vi "Edit_Template_File.vi"(0 "Mode":T3(ring), 7 "Template Filename":path, 11 "Data Files":path[](array[path])) -> (4 "Cancelled":bool, 6 "Template Filename Out":path)   [LabVIEW 2022 SP3]
uses:
  Anemometry/Anemometry Sub Vis/Data_plotting_vis/File_Template_Clus.ctl
  Dispose_Channel.ctl
  Anemometry/Anemometry Sub Vis/Controls/Global_mode.ctl
panel:
  in  "Cancelled":bool
  out "index of element":i32
  in  "Add New Channel Named":bool
  in  "Edit Maths Equation":bool
  out "Current Case Name":string
  in  "Organise Channels":bool
  in  "Add New Channels Fr File":bool
  in  "OK":bool
  in  "Search String":string
  in  "Listbox":i32(listbox)
  out "Channel Name":string
  in  "Cluster":T1 {"Tolerance" min=0.0 format="%#.4f"}
  # "> 20  or  <20  or  =hello   or \n£hello  (not equal to hello)"
  # "<<Characters_to_Match>>  <<Replace_Whole_String_with_this>>"
  # "<<Channel_Name>> contains <<Characters to match>> or\n<<Channel_Name>> does not contain <<Characters to match>>"
  # "<<Channel_Name_A>> + <<Channel_Name_B>> or\nConcatenate <<Channel_Name_A>> and <<Channel_Name_B>>"
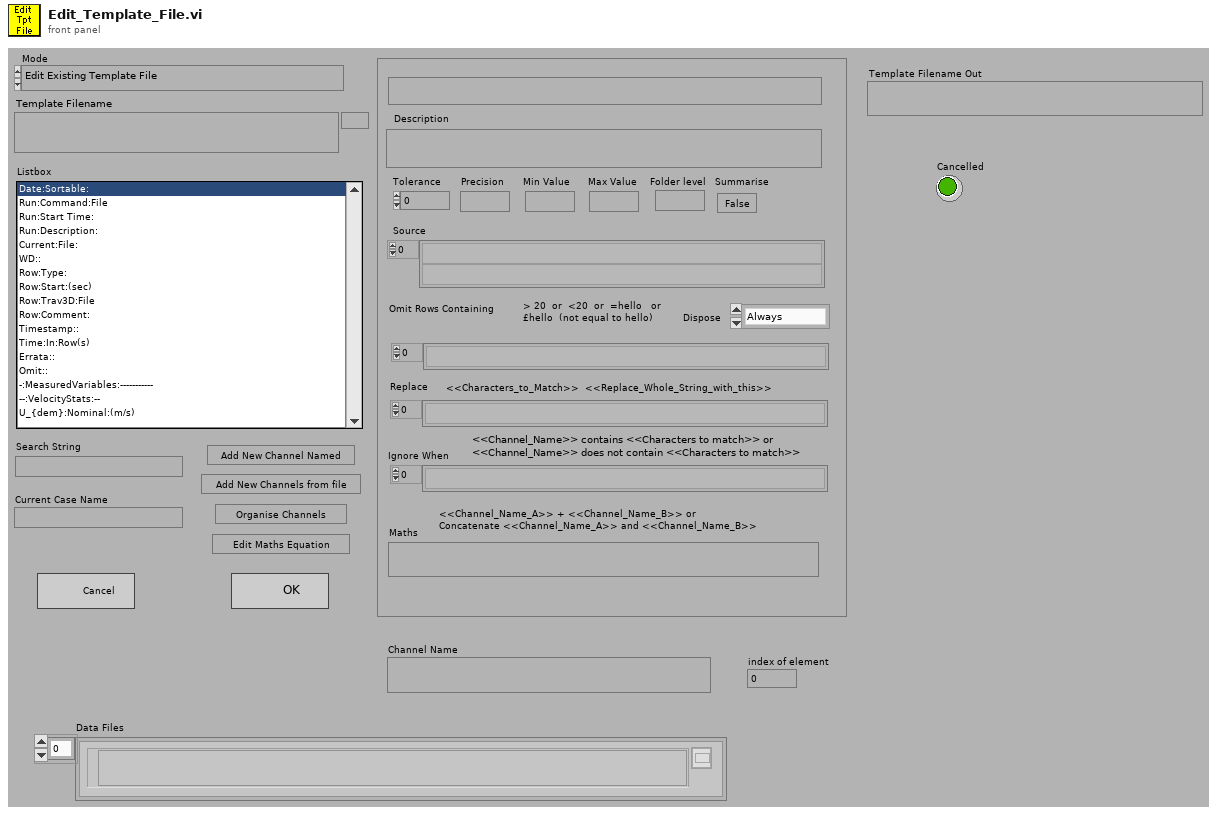
[diagram p1: front panel]
types:
  T1 = typedef "File_Template_Clus.ctl" = cluster{"Template Channel Name":string, "Description":string, "Tolerance":dbl, "Precision":string, "Folder level":string, "Source":string[], "Replace":string[], "Summarise":bool, "Min Value":string, "Maths":string, "Omit Rows Containing":string[], "Ignore When":string[], "Max Value":string, "Dispose":T2}
  T2 = typedef "Dispose_Channel.ctl" = enum16{"Always", "If Blank", "Never"}
  T3 = enum16{"Edit Existing Template File", "Create New Template File"}
  T4 = typedef "Global_mode.ctl" = enum16{"Read Global", "Load Global From File", "Write Global to File"}
  T5 = enum16{"Read Channels From File", "Read Channels from Server"}
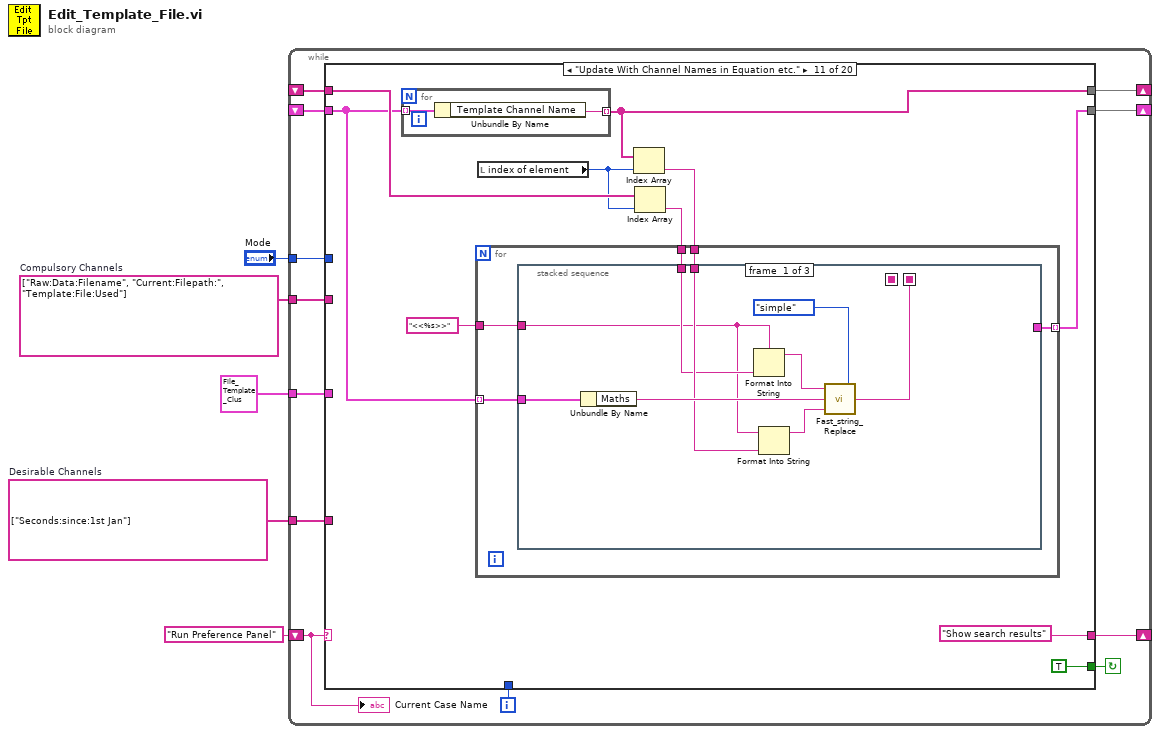
[diagram p0: block diagram]
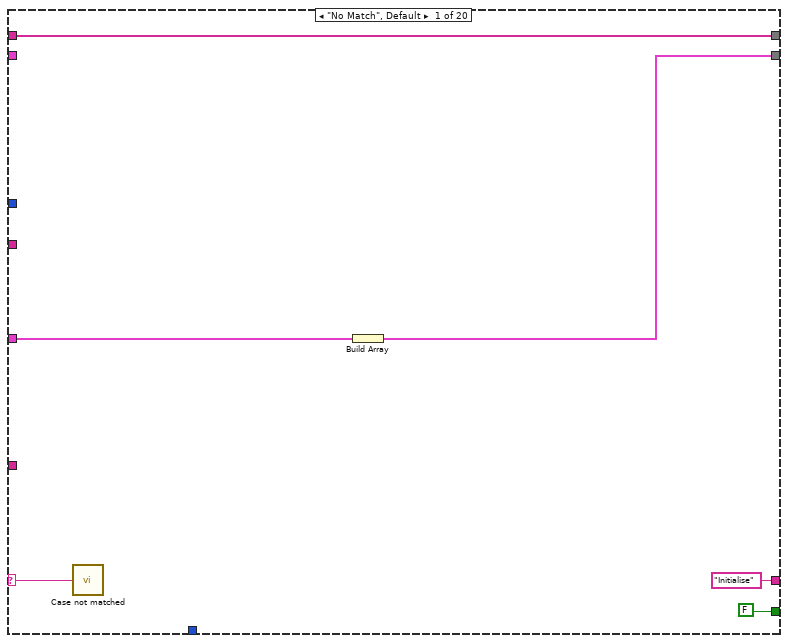
[diagram p2: hidden frame]
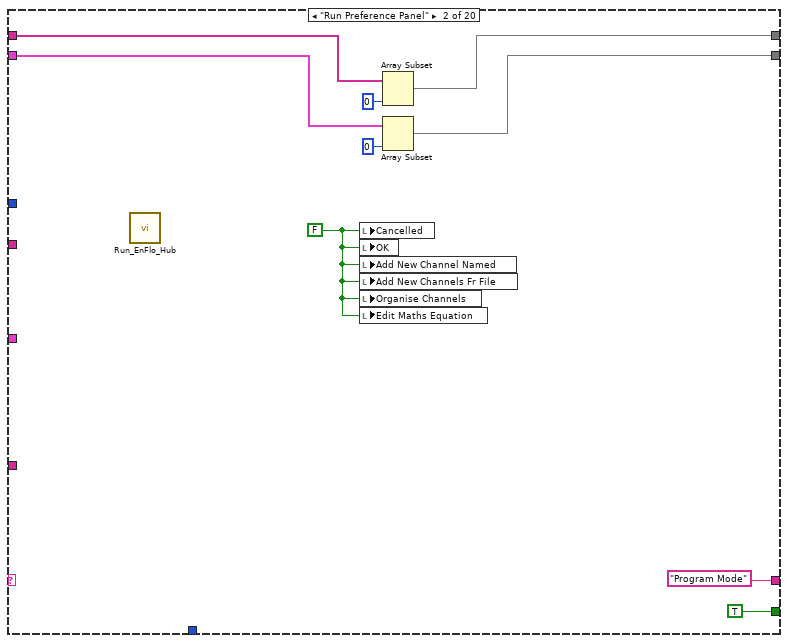
[diagram p3: hidden frame]
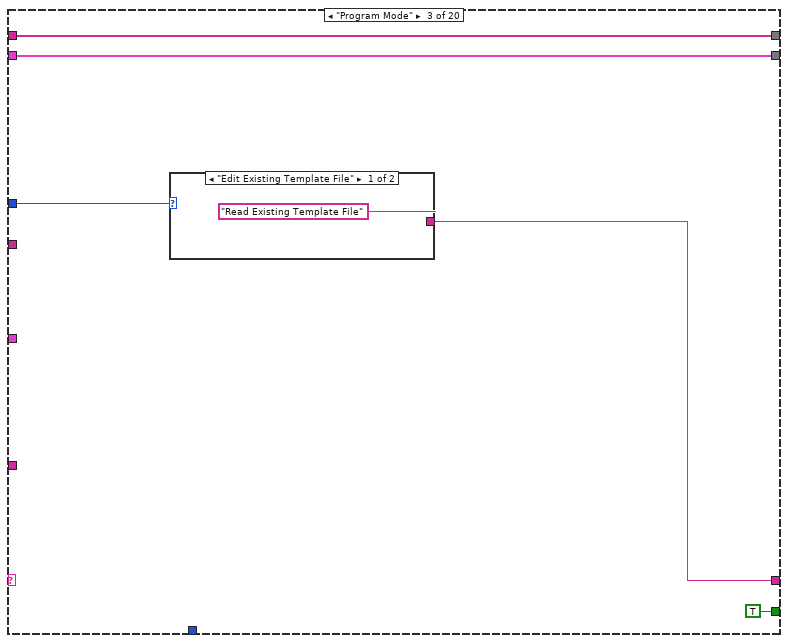
[diagram p4: hidden frame]
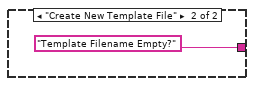
[diagram p5: hidden frame]
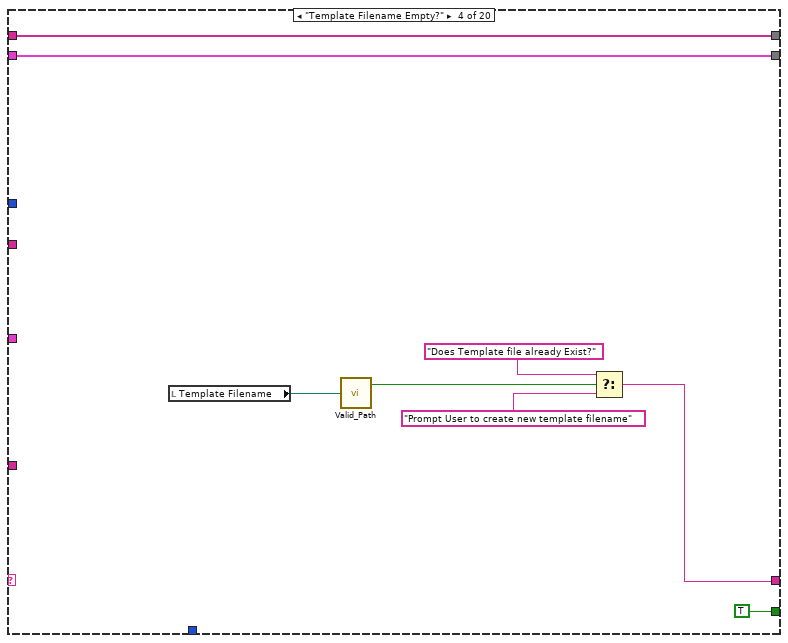
[diagram p6: hidden frame]
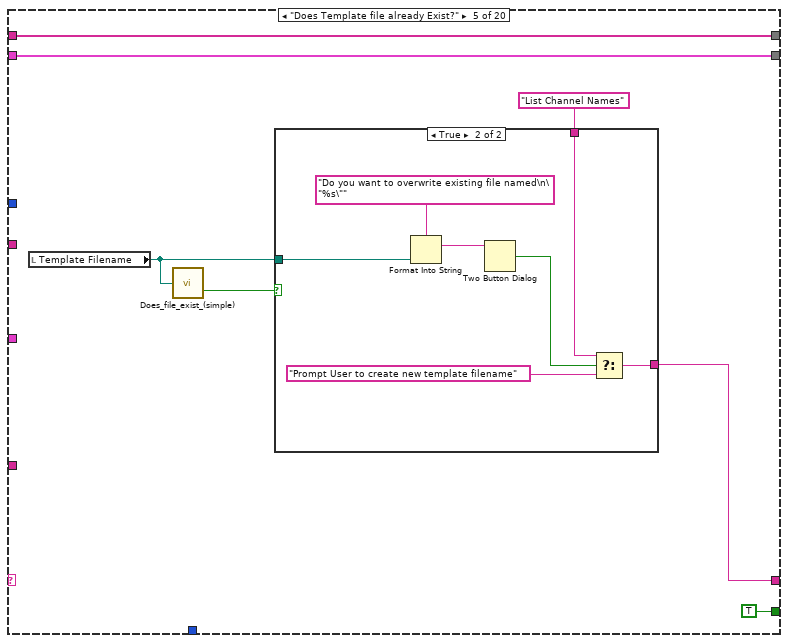
[diagram p7: hidden frame]
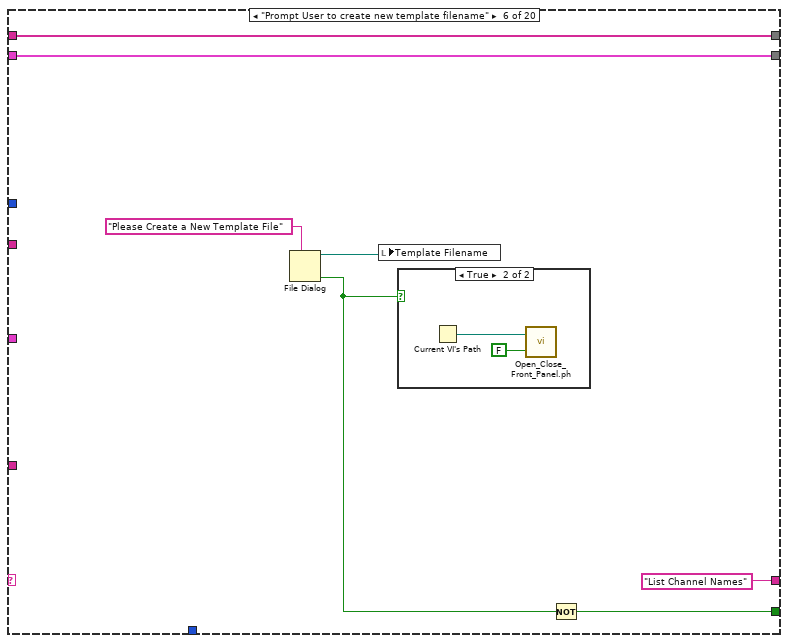
[diagram p9: hidden frame]
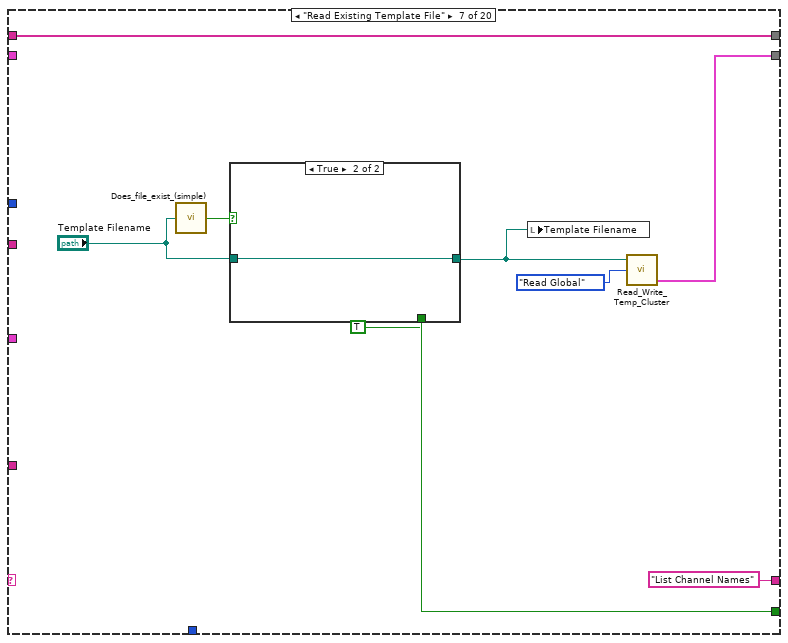
[diagram p11: hidden frame]
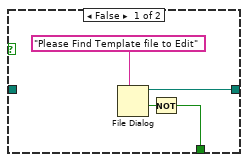
[diagram p12: hidden frame]
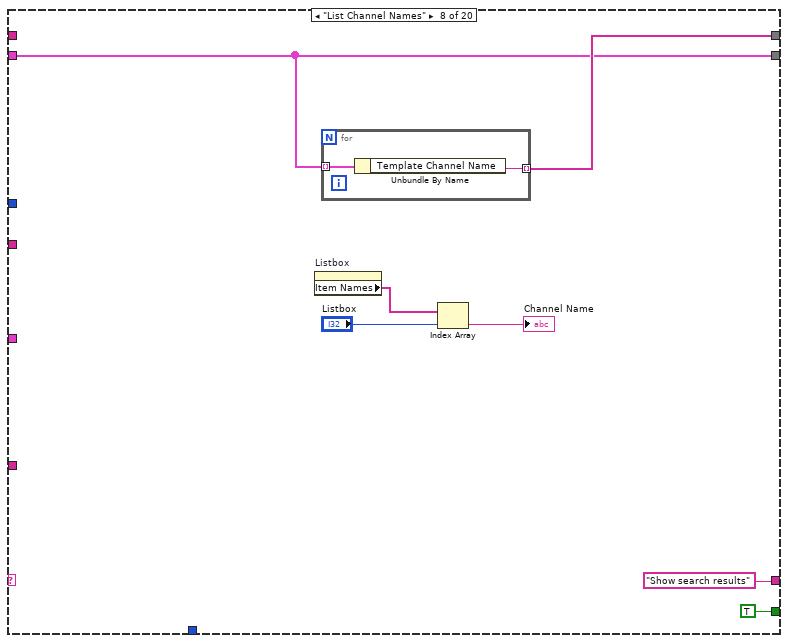
[diagram p13: hidden frame]
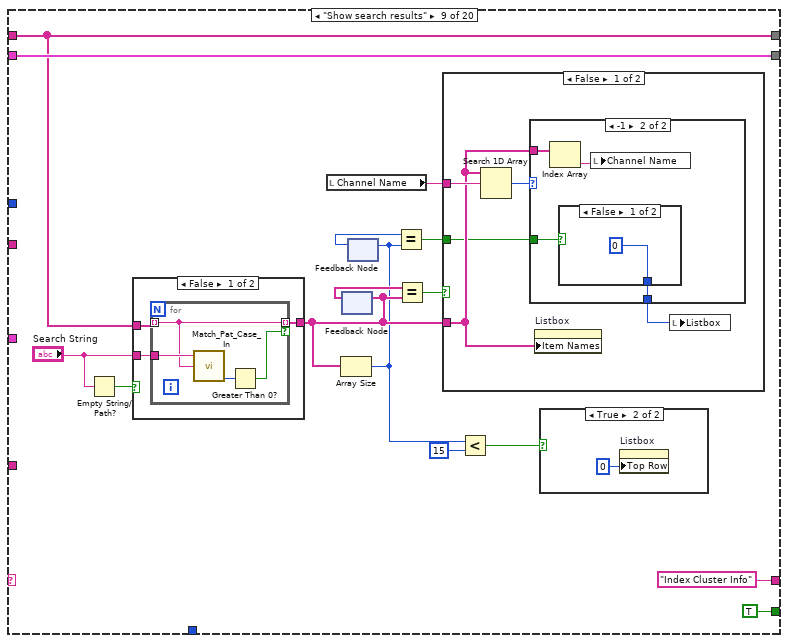
[diagram p14: hidden frame]
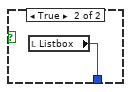
[diagram p17: hidden frame]
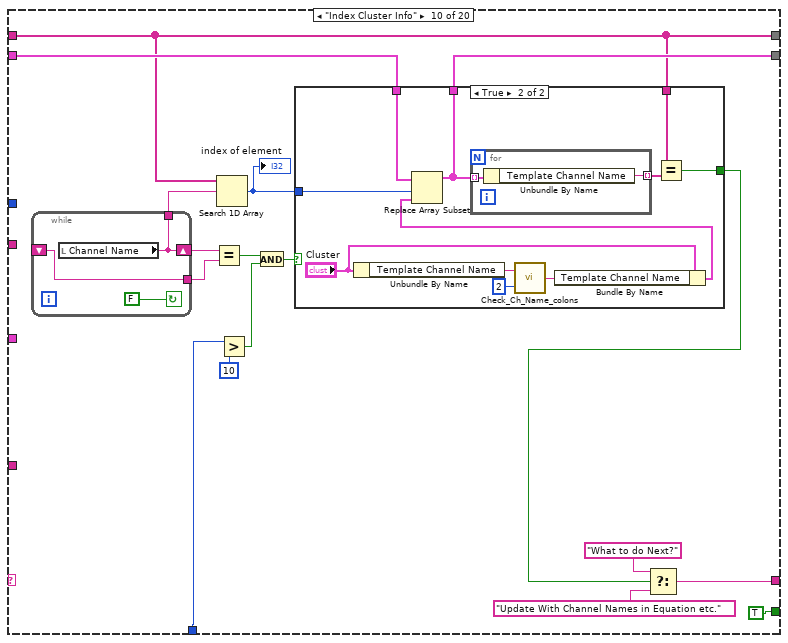
[diagram p20: hidden frame]
diagram:
  w1 = string[] ["Seconds:since:1st Jan"]  # Desirable Channels
  w2 = string[] ["Raw:Data:Filename", "Current:Filepath:", "Template:File:Used"]  # Compulsory Channels
  n1 = while {
    tunnel: T1 {"Template Channel Name"="", "Description"="", "Tolerance"=0.0, "Precision"="", "Folder level"="", "Source"=[], "Replace"=[], "Summarise"=FALSE, "Min Value"="", "Maths"="", "Omit Rows Containing"=[], "Ignore When"=[], "Max Value"="", "Dispose"=enum."Never"} ("Cluster") -> [w11]
    shift-left: _ -> [w12]
    shift-right: [w13] -> _
    tunnel: "Mode" -> [w15]
    shift-left: _ -> [w8]
    shift-right: [w14] -> _
    shift-left: "Run Preference Panel" -> [w10]
    shift-right: [w16] -> _
    tunnel: w2 -> [w7]
    tunnel: w1 -> [w6]
    i -> [w9]
    stop <- w17 continue-if-true
    n2 = case shown="\"Update With Channel Names in Equation etc.\"" w10 {
      selector: w10 -> [w18 _ _ _ _ _ _ _ _ _ _ _ _ _ _ _ _ _ _ _]
      tunnel: [FALSE TRUE TRUE TRUE TRUE w64 w72 TRUE TRUE TRUE TRUE TRUE TRUE TRUE TRUE TRUE TRUE TRUE TRUE FALSE] -> w17
      tunnel: ["Initialise" "Program Mode" w33 w44 w49 "List Channel Names" ("t") "List Channel Names" "Show search results" "Index Cluster Info" w138 "Show search results" "Update cluster info after edit" "Update cluster info after edit" "Update cluster info after edit" "Save Template File" ("t") w301 "Check Tolerance and Precision" "Save Template File" w432 "End" ("t")] -> w16
      tunnel: w15 -> [_ _ w36 _ _ _ _ _ _ _ _ _ _ _ _ _ _ _ _ _]
      tunnel: [w19 w25 w34 w45 w52 w68 w75 w89 w105 w141 w174 w214 w255 w272 w296 w319 w324 w384 w427 w450] -> w14
      tunnel: w8 -> [_ w26 w34 w45 w52 w68 _ w89 w105 w145 w173 w216 w256 w277 w296 w319 w335 w388 w427 w450]
      tunnel: [w21 w28 w35 w46 w53 w69 w74 w91 w104 w137 w175 w215 w257 w279 w298 w320 w331 w385 w436 w451] -> w13
      tunnel: w12 -> [w21 w29 w35 w46 w53 w69 w74 _ w104 w137 w176 w217 w258 w279 w298 w320 w332 w385 w436 w451]
      tunnel: w11 -> [w20 _ _ _ _ _ _ _ _ _ _ w213 _ _ _ _ w322 _ _ _]
      tunnel: w9 -> [_ _ _ _ _ _ _ _ _ w135 _ _ _ _ _ _ _ _ _ _]
      tunnel: w7 -> [_ _ _ _ _ _ _ _ _ _ _ _ _ _ _ _ w328 _ _ _]
      tunnel: w6 -> [_ _ _ _ _ _ _ _ _ _ _ _ _ _ _ _ w325 _ _ _]
      frame "No Match", Default {
        n3 = call "Case not matched.vi"("Case Name not Matched"=w18) -> ()
        n4 = Build Array(w20) -> (w19:T1[])
      }
      frame "Run Preference Panel" {
        w24 = FALSE ("Add channel Fr Results File")
        n5 = call "Run_EnFlo_Hub.vi"() -> ()  [unwired: 1 in, 7 out]
        n6 = local write "Cancelled"(w24) -> ()
        n7 = local write "OK"(w24) -> ()
        n8 = local write "Add New Channel Named"(w24) -> ()
        n9 = local write "Add New Channels Fr File"(w24) -> ()
        n10 = local write "Organise Channels"(w24) -> ()
        n11 = local write "Edit Maths Equation"(w24) -> ()
        n12 = Array Subset(array=w29, length=0 ("Array Length")) -> (w28:string[])  [unwired: 1 in]
        n13 = Array Subset(array=w26, length=0 ("Array Length")) -> (w25:T1[])  [unwired: 1 in]
      }
      frame "Program Mode" {
        n14 = case shown="\"Edit Existing Template File\"" w36 {
          tunnel: ["Read Existing Template File" "Template Filename Empty?"] -> w33
          frame "Edit Existing Template File" {
          }
          frame "Create New Template File" {
          }
        }
      }
      frame "Template Filename Empty?" {
        n15 = local read "Template Filename"() -> (w43:path)
        n16 = call "Valid_Path.vi"("Filename"=w43) -> ("Valid Path?"=w42:bool)
        n17 = Select(t="Does Template file already Exist?", s=w42, f="Prompt User to create new template filename" ("t")) -> (s? t:f=w44:string)
      }
      frame "Does Template file already Exist?" {
        n18 = local read "Template Filename"() -> (w50:path)
        n19 = call "Does_file_exist_(simple).vi"("Pathname"=w50) -> ("exists?"=w51:bool)
        n20 = case shown="True" w51 {
          tunnel: w50 -> [_ w62]
          tunnel: [w55 w57] -> w49
          tunnel: "List Channel Names" ("t") -> [w55 w56]
          frame False {
          }
          frame True {
            n21 = Format Into String(format string="Do you want to overwrite existing file named\n\"%s\"" ("Format String"), w62) -> (resulting string=w60:string)  [unwired: 2 in, 1 out]
            n22 = Two Button Dialog(message=w60) -> (T button?=w58:bool)  [unwired: 2 out]
            n23 = Select(t=w56, s=w58, f="Prompt User to create new template filename") -> (s? t:f=w57:string)
          }
        }
      }
      frame "Prompt User to create new template filename" {
        n24 = File Dialog(7:"Please Create a New Template File" ("prompt")) -> (1:w63:bool, 3:w67:path)  [unwired: 1 in, 7 out]
        n25 = local write "Template Filename"(w67) -> ()
        n26 = case shown="True" w63 {
          frame False {
          }
          frame True {
            n27 = Current VI's Path() -> (path=w71:path)
            n28 = call "Open_Close_Front_Panel.ph.vi"("openWindow (T)"=FALSE ("Front Panel Window:Open"), "VI path"=w71) -> ()  [unwired: 1 in, 1 out]
          }
        }
        n29 = Not(x=w63) -> (.not. x?=w64:bool)
      }
      frame "Read Existing Template File" {
        n30 = call "Does_file_exist_(simple).vi"("Pathname"="Template Filename") -> ("exists?"=w78:bool)
        n31 = case shown="True" w78 {
          tunnel: [w83 w85] -> w73
          tunnel: "Template Filename" -> [_ w85]
          tunnel: [w80 TRUE] -> w72
          frame False {
            n32 = File Dialog(7:"Please Find Template file to Edit" ("prompt")) -> (1:w81:bool, 3:w83:path)  [unwired: 1 in, 7 out]
            n33 = Not(x=w81) -> (.not. x?=w80:bool)
          }
          frame True {
          }
        }
        n34 = local write "Template Filename"(w73) -> ()
        n35 = call "Read_Write_Temp_Cluster.vi"("Mode"=Global_mode."Read Global", "Template File"=w73) -> ("Template Info Array Out"=w75:T1[])  [unwired: 1 in, 2 out]
      }
      frame "List Channel Names" {
        n36 = property on="Listbox" class="LstBox (strict)"() -> ("Item Names"=w88:string[])  [unwired: 2 in, 2 out]
        n37 = for {
          tunnel: w89 -> [w94] mode=indexing
          tunnel: [w93] -> w91 mode=indexing
          n38 = Unbundle By Name(w94) -> ("Template Channel Name"=w93:string)
        }
        n39 = Index Array(array=w88, index="Listbox") -> (element=→"Channel Name":string)
      }
      frame "Show search results" {
        n40 = Empty String/Path?(string/path="Search String") -> (empty?=w107:bool)
        n41 = case shown="False" w107 {
          tunnel: "Search String" -> [w125 _]
          tunnel: w104 -> [w124 w130]
          tunnel: [w123 w130] -> w100
          frame False {
            n42 = for {
              tunnel: w125 -> [w129]
              tunnel: w124 -> [w127] mode=indexing
              tunnel: [w127] -> w123 mode=indexing if=w126
              n43 = call "Match_Pat_Case_In.vi"("String to match"=w129, "String"=w127) -> ("offset past match"=w128:i32)  [unwired: 1 in, 3 out]
              n44 = Greater Than 0?(x=w128) -> (x > 0?=w126:bool)
            }
          }
          frame True {
          }
        }
        n45 = local read "Channel Name"() -> (w101:string)
        n46 = Array Size(array=w100) -> (size(s)=w97:i32)
        n47 = feedback-in #1(w100) -> ()
        n48 = feedback #1() -> (w103:string[])  [unwired: 1 in]
        n49 = feedback #2() -> (w99:i32)  [unwired: 1 in]
        n50 = feedback-in #2(w97) -> ()
        n51 = Equal?(x=w99, y=w97) -> (x = y?=w98:bool)
        n52 = Equal?(x=w103, y=w100) -> (x = y?=w102:bool)
        n53 = case shown="False" w102 {
          tunnel: w100 -> [w113 _]
          tunnel: w101 -> [w115 _]
          tunnel: w98 -> [w112 _]
          frame False {
            n54 = Search 1D Array(1D array=w113, element=w115) -> (index of element=w114:i32)  [unwired: 1 in]
            n55 = case shown="-1" w114 {
              selector: w114 -> [w116 _]
              tunnel: w113 -> [_ w120]
              tunnel: w112 -> [_ w118]
              tunnel: [w116 w117] -> w111
              frame Default {
              }
              frame -1 {
                n56 = Index Array(array=w120) -> (element=w119:string)  [unwired: 1 in]
                n57 = case shown="False" w118 {
                  tunnel: [0 ("Listbox") w122] -> w117
                  frame False {
                  }
                  frame True {
                    n58 = local read "Listbox"() -> (w122:i32)
                  }
                }
                n59 = local write "Channel Name"(w119) -> ()
              }
            }
            n60 = property on="Listbox" class="LstBox (strict)"("Item Names"=w113) -> ()  [unwired: 2 in, 2 out]
            n61 = local write "Listbox"(w111) -> ()
          }
          frame True {
          }
        }
        n62 = Less?(x=w97, y=15) -> (x < y?=w95:bool)
        n63 = case shown="True" w95 {
          frame False {
          }
          frame True {
            n64 = property on="Listbox" class="LstBox (strict)"("Top Row"=0) -> ()  [unwired: 2 in, 2 out]
          }
        }
      }
      frame "Index Cluster Info" {
        n65 = while {
          tunnel: [w149] -> w142
          tunnel: [w150] -> w143
          shift-left: _ -> [w150]
          shift-right: [w149] -> w144
          stop <- FALSE continue-if-true
          n66 = local read "Channel Name"() -> (w149:string)
        }
        n67 = Equal?(x=w144, y=w143) -> (x = y?=w133:bool)
        n68 = Search 1D Array(1D array=w137, element=w142) -> (index of element=w146:i32)  [unwired: 1 out]
        "index of element" <- w146
        n69 = Greater?(x=w135, y=10) -> (0:w132:bool)
        n70 = And(x=w133, y=w132) -> (x .and. y?=w131:bool)
        n71 = case shown="True" w131 {
          tunnel: w146 -> [w154 w164]
          tunnel: w145 -> [w152 w165]
          tunnel: [w152 w161] -> w141
          tunnel: w137 -> [_ w162]
          tunnel: [TRUE w160] -> w136
          frame False {
            n72 = Index Array(array=w152, index=w154) -> (element=w153:T1)
            n73 = local write "Cluster"(w153) -> ()
          }
          frame True {
            n74 = Unbundle By Name("Cluster") -> ("Template Channel Name"=w158:string)
            n75 = call "Check_Ch_Name_colons.vi"("No of Colons"=2, "Ch Name in"=w158) -> ("Ch Name out"=w157:string)
            n76 = Bundle By Name(cluster="Cluster", "Template Channel Name"=w157) -> (w155:T1)
            n77 = Replace Array Subset(array=w165, new element=w155, index=w164) -> (w161:T1[])
            n78 = for {
              tunnel: w161 -> [w167] mode=indexing
              tunnel: [w166] -> w163 mode=indexing
              n79 = Unbundle By Name(w167) -> ("Template Channel Name"=w166:string)
            }
            n80 = Equal?(x=w162, y=w163) -> (x = y?=w160:bool)
          }
        }
        n81 = Select(t="What to do Next?", s=w136, f="Update With Channel Names in Equation etc.") -> (s? t:f=w138:string)
      }
      frame "Update With Channel Names in Equation etc." {
        n82 = for {
          tunnel: w173 -> [w210] mode=indexing
          tunnel: [w209] -> w175 mode=indexing
          n83 = Unbundle By Name(w210) -> ("Template Channel Name"=w209:string)
        }
        n84 = local read "index of element"() -> (w171:i32)
        n85 = Index Array(array=w175, index=w171) -> (element=w169:string)
        n86 = Index Array(array=w176, index=w171) -> (element=w170:string)
        n87 = for {
          tunnel: w173 -> [w180] mode=indexing
          tunnel: w169 -> [w182]
          tunnel: [w179] -> w174 mode=indexing
          tunnel: w170 -> [w181]
          tunnel: "<<%s>>" ("Format String") -> [w178]
          n88 = stacked-sequence {
            seq-local: [w185 _ _] -> [_ _ w208]
            seq-local: [_ w193 _] -> [_ _ w206]
            tunnel: w180 -> [w191 w197 w205]
            tunnel: w182 -> [w189 w195 _]
            tunnel: w181 -> [w186 w194 _]
            tunnel: [_ _ w207] -> w179
            tunnel: w178 -> [w184 w192 _]
            frame #0 {
              n89 = Unbundle By Name(w191) -> ("Maths"=w190:string)
              n90 = Format Into String(format string=w184, w186) -> (resulting string=w187:string)  [unwired: 2 in, 1 out]
              n91 = Format Into String(format string=w184, w189) -> (resulting string=w188:string)  [unwired: 2 in, 1 out]
              n92 = call "Fast_string_Replace.vi"("mode"=enum16{"simple", "regex"}."simple", "Replace match with:"=w188, "Input String"=w190, "matchThis"=w187) -> ("Output String"=w185:string)  [unwired: 1 out]
            }
            frame #1 {
              n93 = Unbundle By Name(w197) -> ("Ignore When"=w196:string[])
              n94 = for {
                tunnel: w196 -> [w204] mode=indexing
                tunnel: w195 -> [w203]
                tunnel: w194 -> [w200]
                tunnel: [w199] -> w193 mode=indexing
                tunnel: w192 -> [w198]
                n95 = Format Into String(format string=w198, w200) -> (resulting string=w201:string)  [unwired: 2 in, 1 out]
                n96 = Format Into String(format string=w198, w203) -> (resulting string=w202:string)  [unwired: 2 in, 1 out]
                n97 = call "Fast_string_Replace.vi"("Replace match with:"=w202, "Input String"=w204, "matchThis"=w201) -> ("Output String"=w199:string)  [unwired: 1 in, 1 out]
              }
            }
            frame #2 {
              n98 = Bundle By Name(cluster=w205, "Maths"=w208, "Ignore When"=w206) -> (w207:T1)
            }
          }
        }
      }
      frame "Select New Channel" {
        n99 = local read "Add New Channel Named"() -> (w212:bool)
        n100 = case shown="False" w212 {
          tunnel: [w223 w227] -> w218
          tunnel: [FALSE ("Add channel Fr Results File") FALSE ("Add channel Fr Results File")] -> w211
          frame False {
            n101 = call "Select_a_Channel.vi"("Mode"=T5."Read Channels From File", "Data Files"="Data Files") -> ("Selected Channel Names"=w223:string[])  [unwired: 1 in, 5 out]
          }
          frame True {
            n102 = call "Input_String_Dialog.vi"("Message to user"="Enter New Channel Name") -> ("Ok Out"=w229:bool, "Output string"=w230:string)  [unwired: 1 in]
            n103 = Build Array(w230) -> (w228:string[])
            n104 = Select(t=w228, s=w229, f=string[] []) -> (s? t:f=w227:string[])
          }
        }
        n105 = for {
          tunnel: w218 -> [w236] mode=indexing
          shift-right: [w234] -> w215
          shift-left: w217 -> [w235]
          shift-right: [w237] -> w214
          shift-left: w216 -> [w238]
          tunnel: w213 -> [w240]
          n106 = Build Array(w236) -> (w243:string[])
          n107 = while {
            tunnel: [w244] -> w233
            tunnel: w236 -> [w246]
            tunnel: w235 -> [w247]
            i -> [w245]
            stop <- w248 continue-if-true
            n108 = case shown="1, Default" w245 {
              selector: w245 -> [_ w251]
              tunnel: [w250 w253] -> w244
              tunnel: w246 -> [w250 w252]
              frame 0 {
              }
              frame 1, Default {
                n109 = Format Into String(format string="%s_DUPLICATE%d" ("Format String"), w252, w251) -> (resulting string=w253:string)  [unwired: 2 in, 1 out]
              }
            }
            n110 = Search 1D Array(1D array=w247, element=w244) -> (index of element=w249:i32)  [unwired: 1 out]
            n111 = Greater Or Equal To 0?(x=w249) -> (x >= 0?=w248:bool)
          }
          n112 = Bundle By Name(cluster=w240, "Template Channel Name"=w233, "Source"=w243, "Summarise"=FALSE ("Bundle Element"), "Dispose"=Dispose_Channel."If Blank", "Tolerance"=1.0 ("Bundle Element")) -> (w239:T1)
          n113 = Build Array (concatenate)(w238, w239) -> (w237:T1[])
          n114 = Build Array (concatenate)(w235, w233) -> (w234:string[])
        }
        n115 = local write "Add New Channel Named"(w211) -> ()
        n116 = local write "Add New Channels Fr File"(w211) -> ()
      }
      frame "Organise Channels" {
        n117 = call "Organise_String_Array.vi"("Input Array"=w258) -> ("Output Array"=w257:string[])
        n118 = for {
          tunnel: w258 -> [w266]
          tunnel: w257 -> [w265] mode=indexing
          tunnel: w256 -> [w263]
          tunnel: [w262] -> w255 mode=indexing
          n119 = Search 1D Array(1D array=w266, element=w265) -> (index of element=w264:i32)  [unwired: 1 out]
          n120 = Index Array(array=w263, index=w264) -> (element=w262:T1)
        }
        n121 = local write "Organise Channels"(FALSE ("Add channel Fr Results File")) -> ()
      }
      frame "Edit Maths Equation" {
        n122 = property on="Listbox" class="LstBox (strict)"() -> ("Item Names"=w269:string[])  [unwired: 2 in, 2 out]
        n123 = local read "Listbox"() -> (w280:i32)
        n124 = Index Array(array=w269, index=w280) -> (element=w278:string)
        n125 = Search 1D Array(1D array=w279, element=w278) -> (index of element=w274:i32)  [unwired: 1 out]
        n126 = Index Array(array=w277, index=w274) -> (element=w273:T1)
        n127 = Unbundle By Name(w273) -> ("Template Channel Name"=w276:string, "Maths"=w275:string)
        n128 = local write "Edit Maths Equation"(FALSE ("Add channel Fr Results File")) -> ()
        n129 = call "Edit_Maths_Equation.vi"("Template Info Array"=w277, "Maths Equation In"=w275, "Channel Name"=w276) -> ("Template Info Array Out"=w271:T1[], "Maths Equation Out"=w268:string)  [unwired: 1 out]
        n130 = Empty String/Path?(string/path=w268) -> (empty?=w267:bool)
        n131 = case shown="False" w267 {
          tunnel: w269 -> [w285 _]
          tunnel: w268 -> [w284 _]
          frame False {
            w286 = TRUE  # Dialog Box (T)
            n132 = call "Do_channel_mathsPLL.vi"("Channel Names"=w285, "Maths Equation"=w284) -> ("Error String"=w290:string)  [unwired: 3 in, 2 out]
            n133 = Empty String/Path?(string/path=w290) -> (empty?=w292:bool)
            n134 = Not(x=w292) -> (.not. x?=w289:bool)
            n135 = Bundle By Name(cluster=errorcluster {"status"=FALSE, "code"=0, "source"=""} ("error in (no error)"), "source"=w290, "status"=w289) -> (w288:errorcluster)
            n136 = call "EnFlo_Error_Handler.vi"("error in (no error)"=w288, "Error Type"="Maths Equation", "Dialog Box (F)"=w286) -> ()  [unwired: 3 out]
          }
          frame True {
          }
        }
        n137 = Bundle By Name(cluster=w273, "Maths"=w268) -> (w270:T1)
        n138 = Replace Array Subset(array=w271, new element=w270, index=w274) -> (w272:T1[])
      }
      frame "Update cluster info after edit" {
        n139 = local read "Channel Name"() -> (w294:string)
        n140 = Search 1D Array(1D array=w298, element=w294) -> (index of element=w297:i32)  [unwired: 1 out]
        n141 = Index Array(array=w296, index=w297) -> (element=w295:T1)
        n142 = local write "Cluster"(w295) -> ()
      }
      frame "What to do Next?" {
        n143 = Select(t="Select New Channel", s="Add New Channels Fr File", f="List Channel Names") -> (s? t:f=w312:string)
        n144 = Select(t="Organise Channels", s="Organise Channels", f=w312) -> (s? t:f=w305:string)
        n145 = Select(t="Edit Maths Equation", s="Edit Maths Equation", f=w305) -> (s? t:f=w307:string)
        n146 = Select(t="Select New Channel", s="Add New Channel Named", f=w307) -> (s? t:f=w306:string)
        n147 = Select(t="Check Template File", s="OK", f=w306) -> (s? t:f=w302:string)
        n148 = Select(t="Close Panel", s="Cancelled", f=w302) -> (s? t:f=w301:string)
        "Cancelled" <- "Cancelled"
      }
      frame "Check Template File" {
        n149 = for {
          tunnel: w335 -> [w381] mode=indexing
          tunnel: [w380] -> w329 mode=indexing
          tunnel: [w379] -> w326 mode=indexing
          n150 = Unbundle By Name(w381) -> ("Template Channel Name"=w382:string)
          n151 = call "Check_Ch_Name_colons.vi"("No of Colons"=2, "Ch Name in"=w382) -> ("Ch Name out"=w379:string)
          n152 = Bundle By Name(cluster=w381, "Template Channel Name"=w379) -> (w380:T1)
        }
        n153 = for {
          tunnel: w328 -> [w360] mode=indexing
          tunnel: w326 -> [w362]
          tunnel: w322 -> [w359]
          tunnel: [w358] -> w330 mode=indexing if=w355
          shift-right: [w356] -> w327
          shift-left: w329 -> [w357]
          n154 = Search 1D Array(1D array=w362, element=w360) -> (index of element=w361:i32)  [unwired: 1 in]
          n155 = case shown="-1" w361 {
            selector: w361 -> [w364 _]
            tunnel: w360 -> [_ w375]
            tunnel: w359 -> [_ w376]
            tunnel: ["" ("Ch Name out") w375] -> w358
            tunnel: w357 -> [w365 w373]
            tunnel: [w363 w372] -> w356
            tunnel: [FALSE TRUE] -> w355
            frame Default {
              n156 = in-place {
                n157 = in-place-array #3(w365, w364) -> (w370:T1)
                n158 = Bundle By Name(cluster=w370, "Dispose"=Dispose_Channel."Never") -> (w369:T1)
                n159 = in-place-array #3(w369) -> (w363:T1[])  [unwired: 1 out]
              }
            }
            frame -1 {
              n160 = Bundle By Name(cluster=w376, "Template Channel Name"=w375, "Dispose"=Dispose_Channel."Never", "Summarise"=FALSE) -> (w374:T1)
              n161 = Build Array (concatenate)(w373, w374) -> (w372:T1[])
            }
          }
        }
        n162 = for {
          tunnel: w325 -> [w341] mode=indexing
          tunnel: w326 -> [w343]
          tunnel: [w340] -> w323 mode=indexing if=w337
          shift-right: [w338] -> w324
          shift-left: w327 -> [w339]
          tunnel: w322 -> [w336]
          n163 = Search 1D Array(1D array=w343, element=w341) -> (index of element=w342:i32)  [unwired: 1 in]
          n164 = case shown="-1" w342 {
            tunnel: w341 -> [_ w352]
            tunnel: ["" ("Ch Name out") w352] -> w340
            tunnel: w339 -> [w344 w350]
            tunnel: [w344 w349] -> w338
            tunnel: [FALSE TRUE] -> w337
            tunnel: w336 -> [_ w347]
            frame Default {
            }
            frame -1 {
              n165 = Bundle By Name(cluster=w347, "Template Channel Name"=w352, "Dispose"=Dispose_Channel."Never", "Summarise"=FALSE) -> (w351:T1)
              n166 = Build Array (concatenate)(w350, w351) -> (w349:T1[])
            }
          }
        }
        n167 = Build Array (concatenate)(w332, w330, w323) -> (w331:string[])
      }
      frame "Check Tolerance and Precision" {
        n168 = for {
          tunnel: w388 -> [w391] mode=indexing
          tunnel: [w392] -> w384 mode=indexing
          n169 = Unbundle By Name(w391) -> ("Tolerance"=w389:dbl, "Precision"=w390:string)
          n170 = Empty String/Path?(string/path=w390) -> (empty?=w393:bool)
          n171 = case shown="False" w393 {
            tunnel: [w397 w425] -> w392
            tunnel: w391 -> [w396 w425]
            tunnel: w390 -> [w400 _]
            tunnel: w389 -> [w395 _]
            frame False {
              n172 = Fract/Exp String To Number(string=w400) -> (number=w394:dbl)  [unwired: 3 in, 1 out]
              n173 = Greater?(x=w395, y=0.7) -> (0:w398:bool)
              n174 = case shown="False" w398 {
                tunnel: [w402 w424] -> w397
                tunnel: w396 -> [w401 w424]
                tunnel: w395 -> [w406 _]
                tunnel: w394 -> [w403 _]
                frame False {
                  n175 = Greater?(x=w406, y=0.07) -> (0:w404:bool)
                  n176 = case shown="True" w404 {
                    tunnel: w403 -> [w410 w417]
                    tunnel: [w408 w419] -> w402
                    tunnel: w401 -> [w407 w418]
                    frame True {
                      n177 = Greater Than 0?(x=w410) -> (x > 0?=w409:bool)
                      n178 = case shown="False" w409 {
                        tunnel: [w412 w414] -> w408
                        tunnel: w407 -> [w413 w414]
                        frame False {
                          n179 = Bundle By Name(cluster=w413, "Precision"="1") -> (w412:T1)
                        }
                        frame True {
                        }
                      }
                    }
                    frame False {
                      n180 = Greater?(x=w417, y=1.0) -> (0:w415:bool)
                      n181 = case shown="False" w415 {
                        tunnel: [w421 w423] -> w419
                        tunnel: w418 -> [w422 w423]
                        frame False {
                          n182 = Bundle By Name(cluster=w422, "Precision"="2") -> (w421:T1)
                        }
                        frame True {
                        }
                      }
                    }
                  }
                }
                frame True {
                }
              }
            }
            frame True {
            }
          }
        }
      }
      frame "Save Template File" {
        n183 = local read "Template Filename"() -> (w428:path)
        "Template Filename Out" <- w428
        n184 = call "Does_file_exist_(simple).vi"("Pathname"=w428) -> ("exists?"=w429:bool)
        n185 = case shown="True" w429 {
          tunnel: w427 -> [_ w440]
          tunnel: [TRUE w438] -> w426
          tunnel: w428 -> [_ w439]
          frame False {
          }
          frame True {
            n186 = call "Read_Write_Temp_Cluster.vi"("Mode"=Global_mode."Read Global", "Template File"=w439) -> ("Template Info Array Out"=w441:T1[])  [unwired: 1 in, 2 out]
            n187 = Not Equal?(x=w441, y=w440) -> (x != y?=w438:bool)
          }
        }
        n188 = local write "Mode"(T3."Edit Existing Template File" ("Mode")) -> ()
        n189 = case shown="True" w426 {
          tunnel: w428 -> [_ w444]
          tunnel: w427 -> [_ w443]
          frame False {
          }
          frame True {
            n190 = call "Read_Write_Temp_Cluster.vi"("Template Info Array"=w443, "Mode"=Global_mode."Write Global to File", "Template File"=w444) -> ()  [unwired: 3 out]
          }
        }
        n191 = local read "OK"() -> (w435:bool)
        n192 = Select(t="Close Panel", s=w435, f="List Channel Names") -> (s? t:f=w432:string)
      }
      frame "Close Panel" {
        n193 = Current VI's Path() -> (path=w447:path)
        n194 = call "Open_Close_Front_Panel.ph.vi"("openWindow (T)"=FALSE ("Front Panel Window:Open"), "VI path"=w447) -> ()  [unwired: 1 in, 1 out]
      }
    }
    "Current Case Name" <- w10
  }
